vi "Get SMO Address.vi"(8 "error in (no error)":errorcluster, 11 "Inst.RP100 in":refnum<class "Inst.RP100.lvclass">) -> (0 "error out":errorcluster, 2 "SMO Address":string, 3 "Inst.RP100 out":refnum<class "Inst.RP100.lvclass">)   [LabVIEW 2019, in "Inst.RP100.lvlib" / "Inst.RP100.lvclass"]
uses:
  Inst.RP100.lvclass
  <userlib>/LevyLab/Instrument Framework/Instrument Types/Strain/Instrument.Strain.lvclass
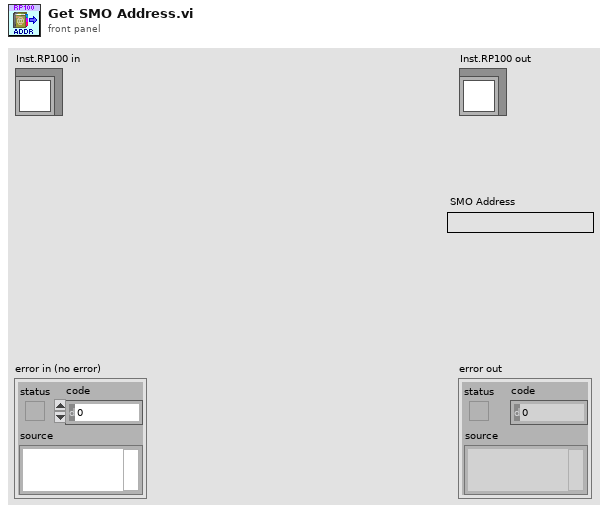
[diagram p1: front panel]
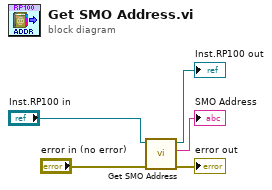
[diagram p0: block diagram]
diagram:
  n1 = call-parent "Get SMO Address.vi"("error in (no error)"="error in (no error)", "Instrument in"="Inst.RP100 in") -> ("error out"=→"error out":errorcluster, "SMO Address"=→"SMO Address":string, "Instrument out"=→"Inst.RP100 out":refnum<class "Inst.RP100.lvclass">)  [unwired: 7 in]
